vi "Destroy.vi"(8 "error in (no error)":errorcluster, 11 "EventMessenger in":refnum<class "EventMessenger.lvclass">) -> (0 "error out":errorcluster)   [LabVIEW 2011, in "Messenging.lvlib" / "EventMessenger.lvclass"]
uses:
  EventMessenger.lvclass
  EventMessenger.lvclass/EventMessenger.ctl
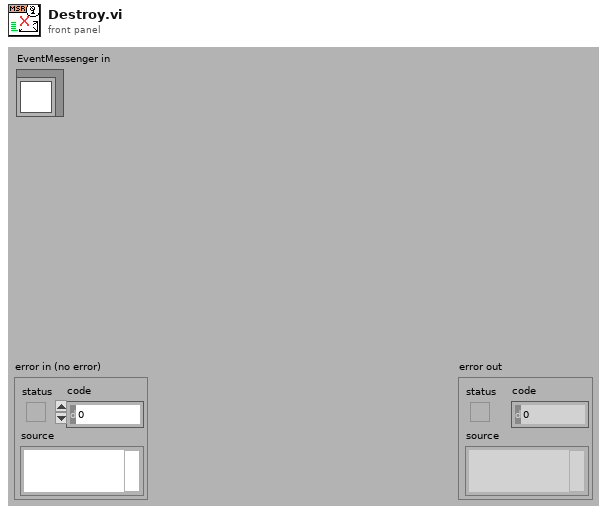
[diagram p1: front panel]
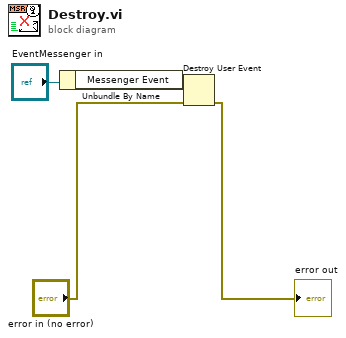
[diagram p0: block diagram]
diagram:
  n1 = Unbundle By Name("EventMessenger in") -> ("Messenger Event"=w3:refnum<user-event>)
  n2 = Destroy User Event(user event=w3, error in="error in (no error)") -> (error out=→"error out":errorcluster)
